vi "Four_terminal_IV_3VoltageAmp_3.1.vi"(0 "Comments":string="SA02610M.20130311\n\nall side gates=0mV\nVbg=-1V\n", 1 "Single IV curve?":bool, 2 "Experiment folder name":string="IV_test", 3 "OSC Configuration":T5(array[cluster])=[{"Signal Type"=enum."Triangle Wave", "DC"=0.00037, "Amplitude"=0.001, "frequency"=0.25, "Phase"=0.0}, {"Signal Type"=enum."Sine Wave", "DC"=0.0, "Amplitude"=0.0, "frequency"=1.0, "Phase"=0.0}, {"Signal Type"=enum."Sine Wave", "DC"=0.0, "Amplitude"=0.0, "frequency"=1.0, "Phase"=0.0}, {"Signal Type"=enum."Sine Wave", "DC"=0.0, "Amplitude"=0.0, "frequency"=1.0, "Phase"=0.0}] {"frequency" format="%0.2p"; "Amplitude" format="%0.2p"; "DC" format="%.2p"}) -> (4 "Two terminal IV":cluster{dbl[], dbl[]}(graph), 5 "I vs V":cluster{dbl[], dbl[]}[](graph), 6 "Temperature (K)":dbl=0.050002, 7 "Field (Oe)":dbl=-0.089, 8 "Connected":string="I-:4\nVbg:3\nV3+:27\nVbg:2\nV1+:28\nI+:1\nV-:5\n")   [LabVIEW 2016]
uses:
  <vilib>/DAQmx/read.llb/DAQmx Read (Analog 2D DBL NChan NSamp).vi
  <vilib>/DAQmx/write.llb/DAQmx Write (Analog 1D Wfm NChan NSamp).vi
  <userlib>/LevyLab/DAQ-Lockin-SubVI/Lockin-4461_MultiChannel - IV 3.0 globals.vi
  SubVI/ITX_Global.vi
  SubVI/PPMS Dashboard.glb.vi
  <resource>/objmgr/daqmx.rc
  <vilib>/DAQmx/configure/timing.llb/DAQmx Timing (Sample Clock).vi
  <vilib>/DAQmx/create/channels.llb/DAQmx Create Channel (AI-Voltage-Basic).vi
  <vilib>/DAQmx/configure/trigger.llb/DAQmx Start Trigger (Digital Edge).vi
  <vilib>/DAQmx/create/channels.llb/DAQmx Create Channel (AO-Voltage-Basic).vi
  <vilib>/measure/NI_MABase.lvlib
panel:
  out "phase log 2":dbl[](array[numeric])
  in  "Tab Control":T1(tab)
  out "Last Scan Image":T2(plugin-control)
  in  "File Path":path=path "C:/Experiments/2011-summer Superconductivity-Spin Hall/Device images/SA02657K_20130302.png"
  in  "PPMS      DR":bool=TRUE
  out "AI Rate":dbl=125000.0 format="%.2p"
  in  "AI Buffer Size (s)":i32=20
  in  "AI Block Size":i32=500000 format="%.0p"
  in  "AI Configuration":T3(array[cluster])=[{"AI.Coupling"=10050, "AI.Max"=10.0, "AI.Min"=-10.0, "Input physical channels"="PXI1Slot2/ai0:1"}, {"AI.Coupling"=10050, "AI.Max"=10.0, "AI.Min"=-10.0, "Input physical channels"="PXI1Slot3/ai0:1"}] {"AI.Coupling" items=["AC"=10045, "DC"=10050, "GND"=10066]}
  in  "AO Configuration":T4(array[cluster])=[{"Output physical channels"="PXI1Slot2/ao0:1", "AO. Max"=1.0, "AO.Min"=-1.0}, {"Output physical channels"="PXI1Slot3/ao0:1", "AO. Max"=10.0, "AO.Min"=-10.0}]
  in  "TIA Gain":dbl=1000000.0
  in  "Voltage Gain":dbl=100.0
  in  "decimating factor":i32=200
  in  "low cutoff freq: fl":dbl=0.1 format="%0.4f"
  in  "Daq settings":u16[](array[ring])=[0, 2, 3, 1] items=["Board 0, AI 0", "Board 0, AI 1", "Board 1, AI 0", "Board 1, AI 1"]
  out "phase log":dbl[](array[numeric])
  out "SamplesAvailable":u32[](array[numeric])=[14, 13]
  out "Sampling information":cluster{"Fs":dbl, "#s":dbl}[](array[cluster])=[{"Fs"=125000.0, "#s"=500000.0}, {"Fs"=125000.0, "#s"=500000.0}]
  out "AO Task":refnum<k21>[](array[refnum])
  out "AI task":refnum<k21>[](array[refnum])
  # "Configurations"
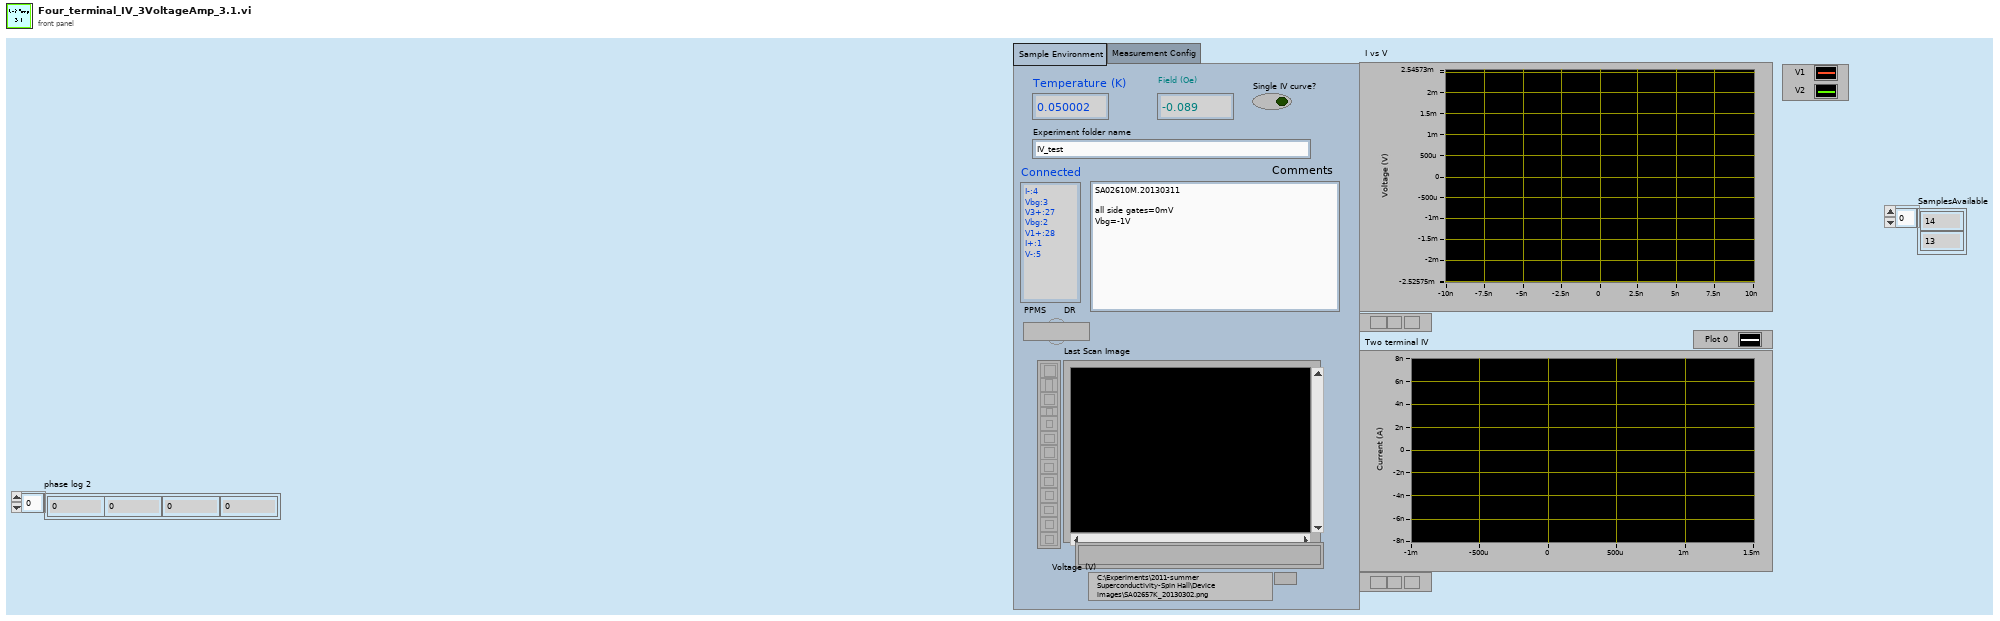
[diagram p1: front panel]
types:
  T1 = enum32{"Sample Environment", "Measurement Config"}
  T2 = typedef "IMAQ Image.ctl" = refnum<image>
  T3 = cluster{"AI.Coupling":i32, "AI.Max":dbl, "AI.Min":dbl, "Input physical channels":tag}[]
  T4 = cluster{"Output physical channels":tag, "AO. Max":dbl, "AO.Min":dbl}[]
  T5 = cluster{"Signal Type":enum16{"Sine Wave", "Triangle Wave", "Square Wave", "Sawtooth Wave"}, "DC":dbl, "Amplitude":dbl, "frequency":dbl, "Phase":dbl}[]
  T6 = cluster{"AI.Coupling":i32, "AI.Max":dbl, "AI.Min":dbl, "Input physical channels":tag}
  T7 = cluster{"Output physical channels":tag, "AO. Max":dbl, "AO.Min":dbl}
  T8 = cluster{"Signal Type":enum16{"Sine Wave", "Triangle Wave", "Square Wave", "Sawtooth Wave"}, "DC":dbl, "Amplitude":dbl, "frequency":dbl, "Phase":dbl}
  T9 = enum16{"Sine Wave", "Triangle Wave", "Square Wave", "Sawtooth Wave"}
  T10 = cluster{"Signal Type":string, "DC":string, "Amplitude":string, "frequency":string, "Phase":string}
  T11 = cluster{"Decimated Array":dbl[], "Decimated Array":dbl[]}[]
  T12 = cluster{"Decimated Array":dbl[], "Decimated Array":dbl[]}
  T13 = enum16{"Sine Wave", "Triangle Wave", "Square Wave", "Sawtooth Wave"}[]
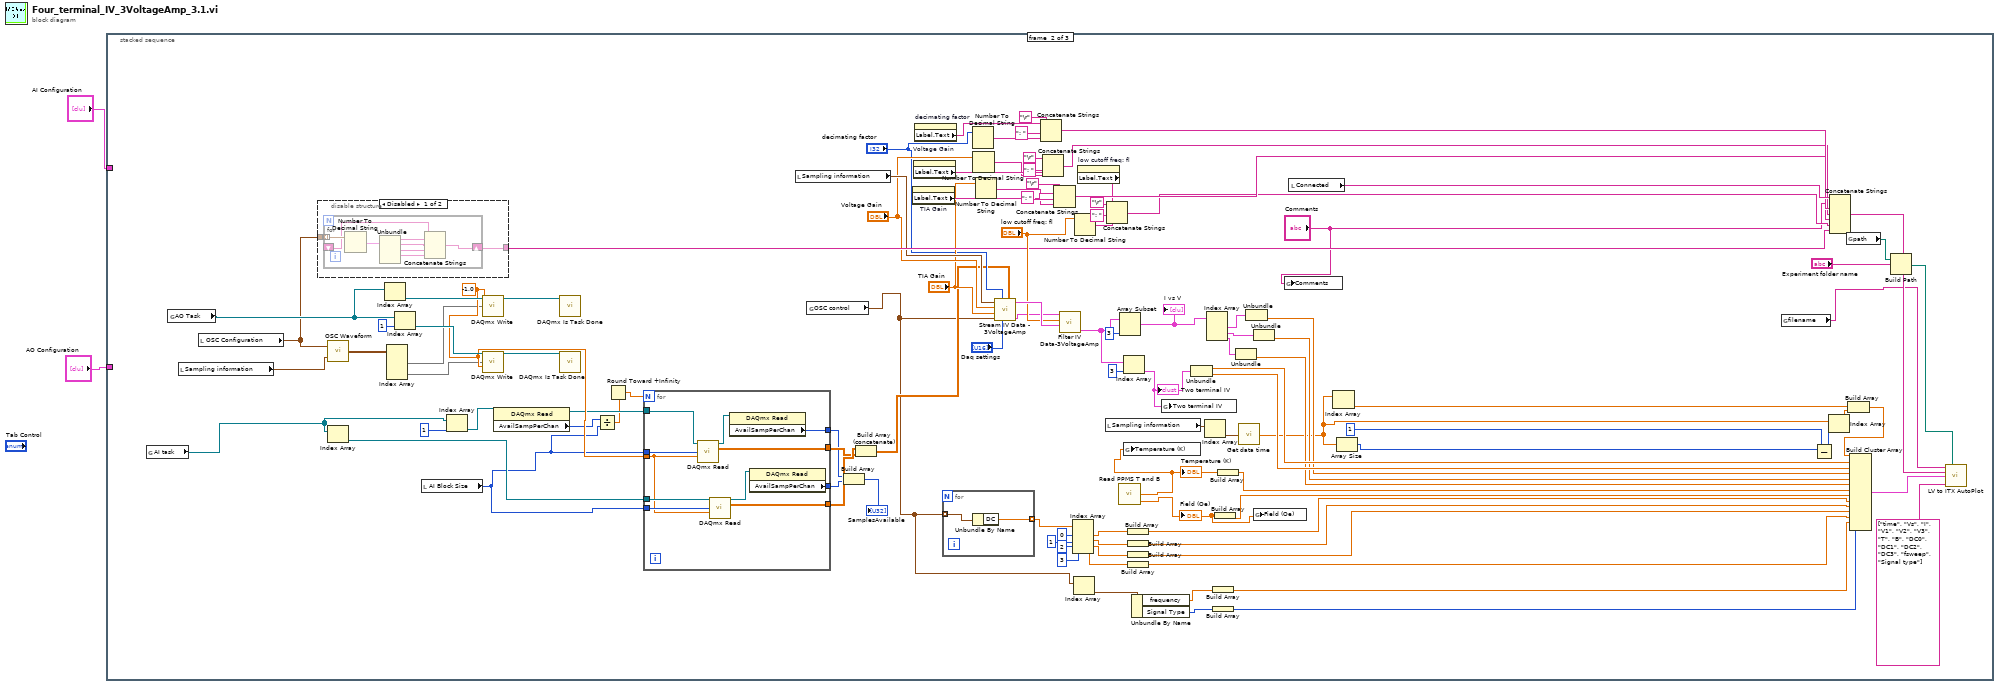
[diagram p0: block diagram]
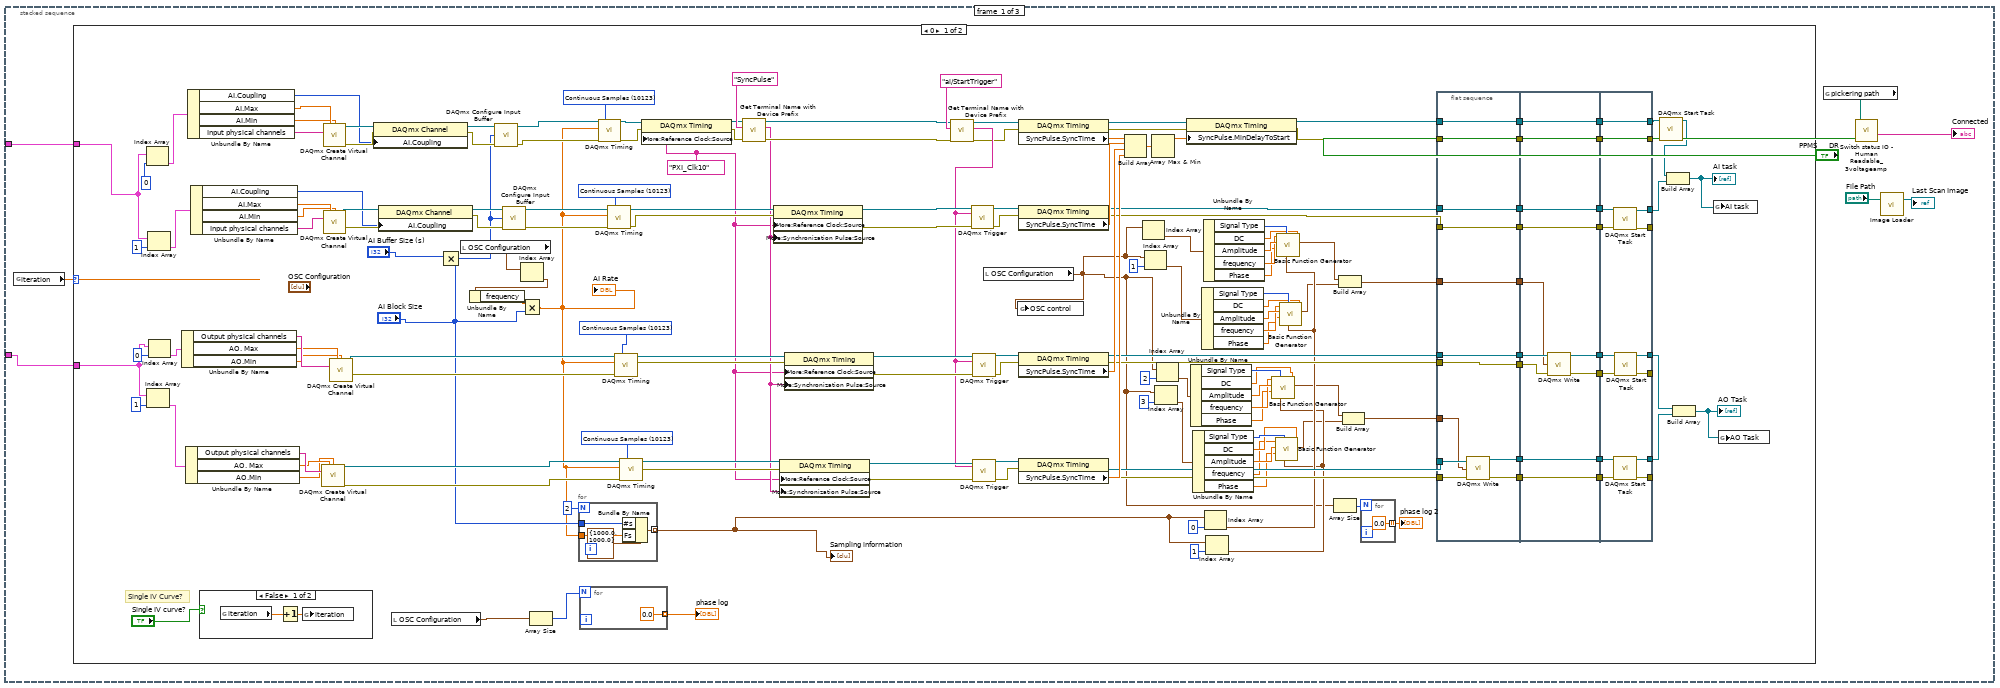
[diagram p2: hidden frame]
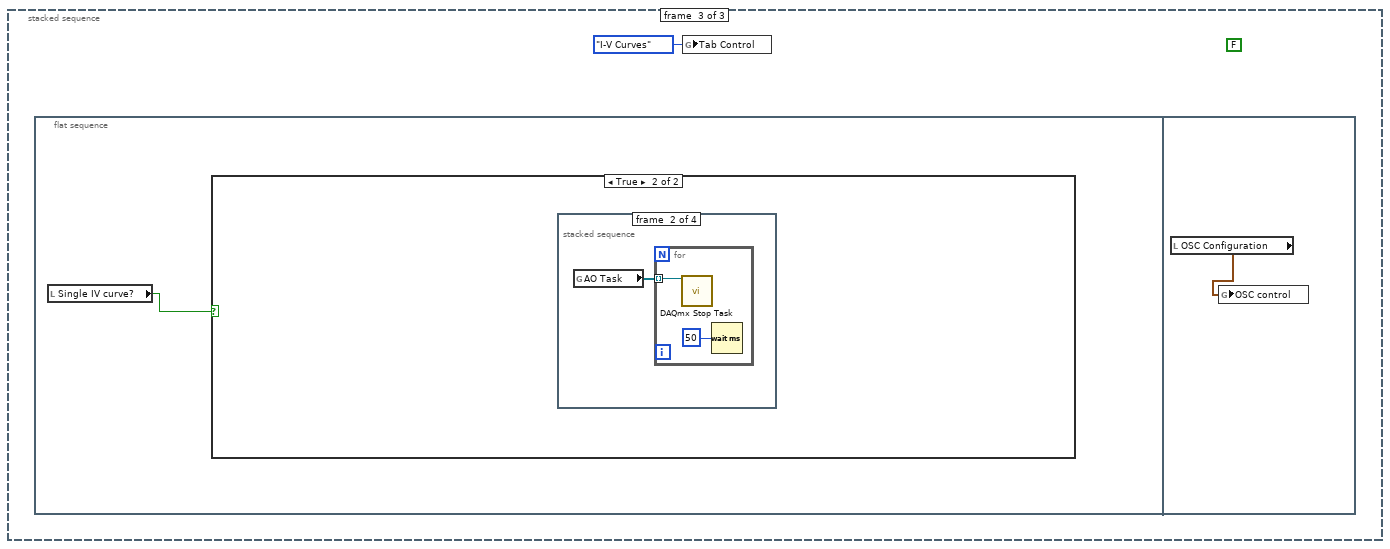
[diagram p6: hidden frame]
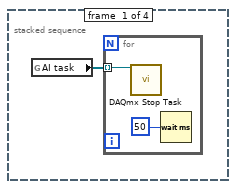
[diagram p8: hidden frame]
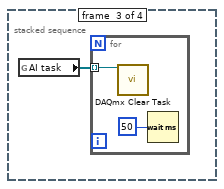
[diagram p9: hidden frame]
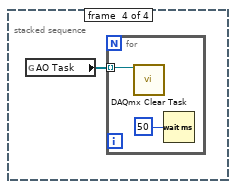
[diagram p10: hidden frame]
diagram:
  n1 = stacked-sequence {
    tunnel: "AI Configuration" -> [w4 _ _]
    tunnel: "AO Configuration" -> [w3 _ _]
    frame #0 {
      n2 = global read "Lockin-4461_MultiChannel - IV 3.0 globals.vi" "iteration"() -> (w10:dbl)
      n3 = case shown="0" w10 {
        tunnel: w4 -> [w20 _]
        tunnel: w3 -> [w19 _]
        frame 0 {
          w81 = tag "PXI_Clk10" ("RefClk.Src")
          w139 = 10123 items=["Finite Samples"=10178, "Continuous Samples"=10123] ("sample mode")
          w140 = 10123 items=["Finite Samples"=10178, "Continuous Samples"=10123] ("sample mode")
          w147 = 10123 items=["Finite Samples"=10178, "Continuous Samples"=10123] ("sample mode")
          w148 = 10123 items=["Finite Samples"=10178, "Continuous Samples"=10123] ("sample mode")
          # "Single IV Curve?"
          n4 = Index Array(array=w20, index=0) -> (element=w152:T6)
          n5 = Index Array(array=w19, index=1) -> (element=w150:T7)
          n6 = Index Array(array=w20, index=1) -> (element=w151:T6)
          n7 = Index Array(array=w19, index=0) -> (element=w149:T7)
          n8 = Unbundle By Name(w149) -> ("Output physical channels"=w90:tag, "AO. Max"=w89:dbl, "AO.Min"=w88:dbl)
          n9 = Unbundle By Name(w150) -> ("Output physical channels"=w87:tag, "AO. Max"=w86:dbl, "AO.Min"=w85:dbl)
          n10 = Unbundle By Name(w152) -> ("AI.Coupling"=w75:i32, "AI.Max"=w95:dbl, "AI.Min"=w94:dbl, "Input physical channels"=w96:tag)
          n11 = Unbundle By Name(w151) -> ("AI.Coupling"=w74:i32, "AI.Max"=w92:dbl, "AI.Min"=w91:dbl, "Input physical channels"=w93:tag)
          n12 = case shown="False" "Single IV curve?" {
            frame False {
              n13 = global read "Lockin-4461_MultiChannel - IV 3.0 globals.vi" "iteration"() -> (w223:dbl)
              n14 = Increment(x=w223) -> (x+1=w222:dbl)
              n15 = global write "Lockin-4461_MultiChannel - IV 3.0 globals.vi" "iteration"(w222) -> ()
            }
            frame True {
            }
          }
          n16 = call-poly <vilib>:"DAQmx Create Virtual Channel.vi"("maximum value"=w86, "minimum value"=w85, "physical channels"=w87) -> ("task out"=w138:refnum<k21>, "error out"=w137:errorcluster)  [unwired: 11 in]
          n17 = call-poly <vilib>:"DAQmx Create Virtual Channel.vi"("maximum value"=w95, "minimum value"=w94, "physical channels"=w96) -> ("task out"=w79:refnum<k21>, "error out"=w78:errorcluster)  [unwired: 11 in]
          n18 = call-poly <vilib>:"DAQmx Create Virtual Channel.vi"("maximum value"=w92, "minimum value"=w91, "physical channels"=w93) -> ("task out"=w77:refnum<k21>, "error out"=w76:errorcluster)  [unwired: 11 in]
          n19 = call-poly <vilib>:"DAQmx Create Virtual Channel.vi"("maximum value"=w89, "minimum value"=w88, "physical channels"=w90) -> ("task out"=w98:refnum<k21>, "error out"=w97:errorcluster)  [unwired: 11 in]
          n20 = property class="DAQmx Channel"(reference=w79, error in=w78, "AI.Coupling"=w75) -> (reference out=w73:refnum<k21>, error out=w72:errorcluster)
          n21 = property class="DAQmx Channel"(reference=w77, error in=w76, "AI.Coupling"=w74) -> (reference out=w71:refnum<k21>, error out=w70:errorcluster)
          n22 = local read "OSC Configuration"() -> (w176:T5)
          n23 = Multiply(x="AI Buffer Size (s)", y="AI Block Size") -> (x*y=w65:i32)
          n24 = local read "OSC Configuration"() -> (w16:T5)
          n25 = call <vilib>:"DAQmx Configure Input Buffer.vi"("task/channels in"=w73, "buffer size (in samples per channel)"=w65, "error in"=w72) -> ("task out"=w69:refnum<k21>, "error out"=w68:errorcluster)  [unwired: 11 in]
          n26 = call <vilib>:"DAQmx Configure Input Buffer.vi"("task/channels in"=w71, "buffer size (in samples per channel)"=w65, "error in"=w70) -> ("task out"=w67:refnum<k21>, "error out"=w66:errorcluster)  [unwired: 11 in]
          n27 = Index Array(array=w16) -> (element=w25:T8)  [unwired: 1 in]
          n28 = Unbundle By Name(w25) -> ("frequency"=w24:dbl)
          n29 = Multiply(x=w24, y="AI Block Size") -> (x*y=w15:dbl)
          "AI Rate" <- w15
          n30 = Array Size(array=w176) -> (size(s)=w178:i32)
          n31 = for {
            N: 2 -> [_]
            tunnel: w15 -> [w183]
            tunnel: "AI Block Size" -> [w182]
            tunnel: [w180] -> w12 mode=indexing
            n32 = Bundle By Name(cluster=cluster{"Fs":dbl, "#s":dbl} {"Fs"=1000.0, "#s"=1000.0} ("sampling info"), "#s"=w182, "Fs"=w183) -> (w180:cluster{"Fs":dbl, "#s":dbl})
          }
          "Sampling information" <- w12
          n33 = for {
            N: w178 -> [_]
            tunnel: [0.0] -> w179 mode=indexing
          }
          "phase log" <- w179
          n34 = call-poly <vilib>:"DAQmx Timing.vi"("task/channels in"=w69, "sample mode"=w148, "rate"=w15, "error in"=w68) -> ("task out"=w142:refnum<k21>, "error out"=w141:errorcluster)  [unwired: 10 in]
          n35 = call-poly <vilib>:"DAQmx Timing.vi"("task/channels in"=w67, "sample mode"=w147, "rate"=w15, "error in"=w66) -> ("task out"=w144:refnum<k21>, "error out"=w143:errorcluster)  [unwired: 10 in]
          n36 = call-poly <vilib>:"DAQmx Timing.vi"("task/channels in"=w98, "sample mode"=w140, "rate"=w15, "error in"=w97) -> ("task out"=w135:refnum<k21>, "error out"=w134:errorcluster)  [unwired: 10 in]
          n37 = call-poly <vilib>:"DAQmx Timing.vi"("task/channels in"=w138, "sample mode"=w139, "rate"=w15, "error in"=w137) -> ("task out"=w136:refnum<k21>, "error out"=w131:errorcluster)  [unwired: 10 in]
          n38 = property class="DAQmx Timing"(reference=w142, error in=w141, "More:Reference Clock:Source"=w81) -> (reference out=w82:refnum<k21>, error out=w80:errorcluster)
          n39 = call "Get Terminal Name with Device Prefix.vi"("error in (no error)"=w80, "Local Terminal Name"="SyncPulse", "task/channels in"=w82) -> ("error out"=w124:errorcluster, "Terminal Name with Device Prefix"=w83:tag, "task out"=w125:refnum<k21>)  [unwired: 6 in]
          n40 = property class="DAQmx Timing"(reference=w144, error in=w143, "More:Reference Clock:Source"=w81, "More:Synchronization Pulse:Source"=w83) -> (reference out=w146:refnum<k21>, error out=w145:errorcluster)
          n41 = property class="DAQmx Timing"(reference=w136, error in=w131, "More:Reference Clock:Source"=w81, "More:Synchronization Pulse:Source"=w83) -> (reference out=w128:refnum<k21>, error out=w127:errorcluster)
          n42 = property class="DAQmx Timing"(reference=w135, error in=w134, "More:Reference Clock:Source"=w81, "More:Synchronization Pulse:Source"=w83) -> (reference out=w130:refnum<k21>, error out=w129:errorcluster)
          n43 = call "Get Terminal Name with Device Prefix.vi"("error in (no error)"=w124, "Local Terminal Name"="ai/StartTrigger", "task/channels in"=w125) -> ("error out"=w121:errorcluster, "Terminal Name with Device Prefix"=w123:tag, "task out"=w122:refnum<k21>)  [unwired: 6 in]
          n44 = call-poly <vilib>:"DAQmx Trigger.vi"("task/channels in"=w146, "source"=w123, "error in"=w145) -> ("task out"=w117:refnum<k21>, "error out"=w118:errorcluster)  [unwired: 11 in]
          n45 = call-poly <vilib>:"DAQmx Trigger.vi"("task/channels in"=w130, "source"=w123, "error in"=w129) -> ("task out"=w115:refnum<k21>, "error out"=w116:errorcluster)  [unwired: 11 in]
          n46 = call-poly <vilib>:"DAQmx Trigger.vi"("task/channels in"=w128, "source"=w123, "error in"=w127) -> ("task out"=w120:refnum<k21>, "error out"=w119:errorcluster)  [unwired: 11 in]
          n47 = local read "OSC Configuration"() -> (w11:T5)
          n48 = global write "Lockin-4461_MultiChannel - IV 3.0 globals.vi" "OSC control"(w11) -> ()
          n49 = property class="DAQmx Timing"(reference=w122, error in=w121) -> (reference out=w112:refnum<k21>, error out=w113:errorcluster, "SyncPulse.SyncTime"=w114:dbl)
          n50 = property class="DAQmx Timing"(reference=w117, error in=w118) -> (reference out=w103:refnum<k21>, error out=w104:errorcluster, "SyncPulse.SyncTime"=w109:dbl)
          n51 = property class="DAQmx Timing"(reference=w115, error in=w116) -> (reference out=w101:refnum<k21>, error out=w102:errorcluster, "SyncPulse.SyncTime"=w108:dbl)
          n52 = property class="DAQmx Timing"(reference=w120, error in=w119) -> (reference out=w99:refnum<k21>, error out=w100:errorcluster, "SyncPulse.SyncTime"=w107:dbl)
          n53 = Build Array(w114, w109, w108, w107) -> (w111:dbl[])
          n54 = Index Array(array=w11) -> (element=w62:T8)  [unwired: 1 in]
          n55 = Index Array(array=w11, index=1) -> (element=w61:T8)
          n56 = Array Max & Min(array=w111) -> (max value=w110:dbl)  [unwired: 3 out]
          n57 = Index Array(array=w11, index=3) -> (element=w60:T8)
          n58 = Index Array(array=w11, index=2) -> (element=w63:T8)
          n59 = property class="DAQmx Timing"(reference=w112, error in=w113, "SyncPulse.MinDelayToStart"=w110) -> (reference out=w105:refnum<k21>, error out=w106:errorcluster)
          n60 = Unbundle By Name(w63) -> ("Signal Type"=w49:T9, "DC"=w48:dbl, "Amplitude"=w47:dbl, "frequency"=w46:dbl, "Phase"=w45:dbl)
          n61 = Unbundle By Name(w60) -> ("Signal Type"=w44:T9, "DC"=w43:dbl, "Amplitude"=w42:dbl, "frequency"=w41:dbl, "Phase"=w40:dbl)
          n62 = Unbundle By Name(w61) -> ("Signal Type"=w54:T9, "DC"=w53:dbl, "Amplitude"=w52:dbl, "frequency"=w51:dbl, "Phase"=w50:dbl)
          n63 = Unbundle By Name(w62) -> ("Signal Type"=w59:T9, "DC"=w58:dbl, "Amplitude"=w57:dbl, "frequency"=w56:dbl, "Phase"=w55:dbl)
          n64 = Index Array(array=w12, index=0) -> (element=w37:cluster{"Fs":dbl, "#s":dbl})
          n65 = Index Array(array=w12, index=1) -> (element=w36:cluster{"Fs":dbl, "#s":dbl})
          n66 = call <vilib>:"Basic Function Generator.vi"("offset"=w48, "sampling info"=w36, "signal type"=w49, "phase"=w45, "amplitude"=w47, "frequency"=w46) -> ("signal out"=w32:waveform(dbl))  [unwired: 3 in, 2 out]
          n67 = call <vilib>:"Basic Function Generator.vi"("offset"=w43, "sampling info"=w36, "signal type"=w44, "phase"=w40, "amplitude"=w42, "frequency"=w41) -> ("signal out"=w31:waveform(dbl))  [unwired: 3 in, 2 out]
          n68 = call <vilib>:"Basic Function Generator.vi"("offset"=w58, "sampling info"=w37, "signal type"=w59, "phase"=w55, "amplitude"=w57, "frequency"=w56) -> ("signal out"=w35:waveform(dbl))  [unwired: 3 in, 2 out]
          n69 = call <vilib>:"Basic Function Generator.vi"("offset"=w53, "sampling info"=w37, "signal type"=w54, "phase"=w50, "amplitude"=w52, "frequency"=w51) -> ("signal out"=w34:waveform(dbl))  [unwired: 3 in, 2 out]
          n70 = Array Size(array=w11) -> (size(s)=w157:i32)
          n71 = Build Array(w35, w34) -> (w33:waveform(dbl)[])
          n72 = Build Array(w32, w31) -> (w30:waveform(dbl)[])
          n73 = for {
            N: w157 -> [_]
            tunnel: [0.0] -> w158 mode=indexing
          }
          "phase log 2" <- w158
          n74 = flat-sequence {
            tunnel: w106 -> [w192]
            tunnel: w105 -> [w193]
            tunnel: w104 -> [w194]
            tunnel: w103 -> [w195]
            tunnel: [w195] -> w175
            tunnel: [w194] -> w174
            tunnel: [w193] -> w173
            tunnel: [w192] -> w172
            tunnel: [w191] -> w171
            tunnel: w102 -> [w191]
            tunnel: [w190] -> w170
            tunnel: w101 -> [w190]
            tunnel: w100 -> [w189]
            tunnel: w99 -> [w188]
            tunnel: [w187] -> w169
            tunnel: [w186] -> w168
            tunnel: w33 -> [w185]
            tunnel: [w185] -> w167
            tunnel: w30 -> [w184]
            tunnel: [w206] -> w166
            tunnel: [w205] -> w165
            tunnel: [w204] -> w164
            tunnel: [w203] -> w163
            tunnel: w175 -> [w206]
            tunnel: w174 -> [w205]
            tunnel: w173 -> [w204]
            tunnel: w172 -> [w203]
            tunnel: w171 -> [w202]
            tunnel: w170 -> [w201]
            tunnel: [w200] -> w162
            tunnel: w169 -> [w200]
            tunnel: [w199] -> w161
            tunnel: w168 -> [w199]
            tunnel: [w198] -> w160
            tunnel: [w197] -> w159
            tunnel: w167 -> [w196]
            tunnel: [w213] -> _
            tunnel: [w214] -> w27
            tunnel: [w215] -> _
            tunnel: [w216] -> w26
            tunnel: [w217] -> _
            tunnel: [w219] -> w28
            tunnel: [w212] -> w133
            tunnel: [w211] -> w132
            tunnel: w166 -> [w220]
            tunnel: w165 -> [w218]
            tunnel: w164 -> [w212]
            tunnel: w163 -> [w211]
            tunnel: w162 -> [w210]
            tunnel: w161 -> [w209]
            tunnel: w160 -> [w208]
            tunnel: w159 -> [w207]
            frame #0 {
              n75 = call-poly <vilib>:"DAQmx Write.vi"("task/channels in"=w188, "data"=w184, "error in"=w189) -> ("task out"=w186:refnum<k21>, "error out"=w187:errorcluster)  [unwired: 10 in, 1 out]
            }
            frame #1 {
              n76 = call-poly <vilib>:"DAQmx Write.vi"("task/channels in"=w201, "data"=w196, "error in"=w202) -> ("task out"=w197:refnum<k21>, "error out"=w198:errorcluster)  [unwired: 10 in, 1 out]
            }
            frame #2 {
              n77 = call <vilib>:"DAQmx Start Task.vi"("task/channels in"=w220, "error in"=w218) -> ("task out"=w219:refnum<k21>, "error out"=w217:errorcluster)  [unwired: 12 in]
              n78 = call <vilib>:"DAQmx Start Task.vi"("task/channels in"=w209, "error in"=w210) -> ("task out"=w216:refnum<k21>, "error out"=w215:errorcluster)  [unwired: 12 in]
              n79 = call <vilib>:"DAQmx Start Task.vi"("task/channels in"=w207, "error in"=w208) -> ("task out"=w214:refnum<k21>, "error out"=w213:errorcluster)  [unwired: 12 in]
            }
          }
          n80 = call <vilib>:"DAQmx Start Task.vi"("task/channels in"=w133, "error in"=w132) -> ("task out"=w29:refnum<k21>)  [unwired: 12 in, 1 out]
          n81 = Build Array(w29, w28) -> (w14:refnum<k21>[])
          "AI task" <- w14
          n82 = Build Array(w27, w26) -> (w13:refnum<k21>[])
          "AO Task" <- w13
          n83 = global write "Lockin-4461_MultiChannel - IV 3.0 globals.vi" "AI task"(w14) -> ()
          n84 = global write "Lockin-4461_MultiChannel - IV 3.0 globals.vi" "AO Task"(w13) -> ()
        }
        frame 1, Default {
        }
      }
      n85 = global read "ITX_Global.vi" "pickering path"() -> (w7:path)
      n86 = call <userlib>:"Switch status IO - Human Readable_3voltageamp.vi"("PPMS      DR"="PPMS      DR", "Switch status"=w7) -> ("String"=→"Connected":string)  [unwired: 2 in]
      n87 = call "Image Loader.vi"("File Path"="File Path") -> ("Last Scan Image"=→"Last Scan Image":T2)  [unwired: 2 in]
    }
    frame #1 {
      w321 = -1.0 ("timeout")
      n88 = global read "Lockin-4461_MultiChannel - IV 3.0 globals.vi" "AI task"() -> (w332:refnum<k21>[])
      n89 = global read "Lockin-4461_MultiChannel - IV 3.0 globals.vi" "AO Task"() -> (w292:refnum<k21>[])
      n90 = local read "Sampling information"() -> (w334:cluster{"Fs":dbl, "#s":dbl}[])
      n91 = local read "OSC Configuration"() -> (w227:T5)
      n92 = disable-structure shown="Disabled" {
        disable-tunnel: w227 -> [w349 _]
        disable-tunnel: [w348 _] -> w318
        frame Disabled {
          n93 = for {
            tunnel: w349 -> [w357] mode=indexing
            shift-right: [w351] -> w348
            shift-left: _ -> [w350]
            n94 = Number To Decimal String(number=w357) -> (decimal integer string=w356:T10)  [unwired: 1 in]
            n95 = Unbundle(w356) -> ("Signal Type"=w355:string, "DC"=w354:string, "Amplitude"=w353:string, "frequency"=w352:string)  [unwired: 1 out]
            n96 = Concatenate Strings(w350, w355, w354, w353, w352) -> (w351:string)
          }
        }
        frame Enabled {
        }
      }
      n97 = call "OSC Waveform.vi"("Sampling information"=w334, "OSC Configuration"=w227) -> ("OSC Waveforms"=w327:waveform(dbl)[][])
      n98 = Index Array(array=w332) -> (element=w331:refnum<k21>)  [unwired: 1 in]
      n99 = Index Array(array=w292) -> (element=w326:refnum<k21>)  [unwired: 1 in]
      n100 = Index Array(array=w327) -> (element #1=w290:waveform(dbl)[], element #2=w291:waveform(dbl)[])  [unwired: 4 in]
      n101 = Index Array(array=w292, index=1) -> (element=w324:refnum<k21>)
      n102 = local read "AI Block Size"() -> (w229:i32)
      n103 = Index Array(array=w332, index=1) -> (element=w238:refnum<k21>)
      n104 = call-poly <vilib>:"DAQmx Write.vi"("task/channels in"=w326, "data"=w290, "timeout"=w321) -> ("task out"=w329:refnum<k21>)  [unwired: 10 in, 2 out]
      n105 = call-poly <vilib>:"DAQmx Write.vi"("task/channels in"=w324, "data"=w291, "timeout"=w321) -> ("task out"=w328:refnum<k21>)  [unwired: 10 in, 2 out]
      n106 = property class="DAQmx Read"(reference=w238) -> (reference out=w237:refnum<k21>, "AvailSampPerChan"=w236:u32)  [unwired: 1 in, 1 out]
      n107 = call <vilib>:"DAQmx Is Task Done.vi"("task/channels in"=w329) -> ()  [unwired: 12 in, 3 out]
      n108 = call <vilib>:"DAQmx Is Task Done.vi"("task/channels in"=w328) -> ()  [unwired: 12 in, 3 out]
      n109 = Divide(x=w236, y=w229) -> (x/y=w235:dbl)
      n110 = Round Toward +Infinity(x=w235) -> (ceil(x): smallest int >= x=w228:dbl)
      n111 = for {
        N: w228 -> [_]
        tunnel: w331 -> [w345]
        tunnel: [w344] -> w323
        tunnel: w229 -> [w343]
        tunnel: [w342] -> w322
        tunnel: w321 -> [w341]
        tunnel: w237 -> [w340]
        tunnel: w229 -> [w339]
        tunnel: [w336] -> w234
        tunnel: [w335] -> w233
        n112 = call-poly <vilib>:"DAQmx Read.vi"("task/channels in"=w340, "number of samples per channel"=w339, "timeout"=w341) -> ("task out"=w338:refnum<k21>, "data"=w342:dbl[][])  [unwired: 10 in, 1 out]
        n113 = call-poly <vilib>:"DAQmx Read.vi"("task/channels in"=w345, "number of samples per channel"=w343, "timeout"=w341) -> ("task out"=w337:refnum<k21>, "data"=w344:dbl[][])  [unwired: 10 in, 1 out]
        n114 = property class="DAQmx Read"(reference=w338) -> ("AvailSampPerChan"=w336:u32)  [unwired: 1 in, 2 out]
        n115 = property class="DAQmx Read"(reference=w337) -> ("AvailSampPerChan"=w335:u32)  [unwired: 1 in, 2 out]
      }
      n116 = local read "Sampling information"() -> (w297:cluster{"Fs":dbl, "#s":dbl}[])
      n117 = global read "Lockin-4461_MultiChannel - IV 3.0 globals.vi" "OSC control"() -> (w226:T5)
      n118 = Build Array(w234, w233) -> (→"SamplesAvailable":u32[])
      n119 = Build Array (concatenate)(w323, w322) -> (w293:dbl[][])
      n120 = property on="TIA Gain" class="DigNum (strict)"() -> ("Label.Text"=w304:string)  [unwired: 2 in, 2 out]
      n121 = property on="Voltage Gain" class="DigNum (strict)"() -> ("Label.Text"=w311:string)  [unwired: 2 in, 2 out]
      n122 = property on="decimating factor" class="DigNum (strict)"() -> ("Label.Text"=w307:string)  [unwired: 2 in, 2 out]
      n123 = for {
        tunnel: w226 -> [w347] mode=indexing
        tunnel: [w346] -> w262 mode=indexing
        n124 = Unbundle By Name(w347) -> ("DC"=w346:dbl)
      }
      n125 = Number To Decimal String(number="decimating factor") -> (decimal integer string=w306:string)  [unwired: 1 in]
      n126 = Number To Decimal String(number="Voltage Gain") -> (decimal integer string=w310:string)  [unwired: 1 in]
      n127 = Number To Decimal String(number="TIA Gain") -> (decimal integer string=w303:string)  [unwired: 1 in]
      n128 = call "Stream IV Data - 3VoltageAmp.vi"("Input signal"=w293, "Daq settings"="Daq settings", "decimating factor"="decimating factor", "OSC Configuration"=w226, "TIA Gain"="TIA Gain", "Voltage Gain"="Voltage Gain", "Sampling information"=w297) -> ("Four terminal IVs"=w286:T11, "Two terminal IV"=w333:T12)  [unwired: 3 in]
      n129 = Concatenate Strings("\r" ("string"), w307, ": " ("string"), w306) -> (w317:string)
      n130 = Concatenate Strings("\r" ("string"), w311, ": " ("string"), w310) -> (w316:string)
      n131 = Concatenate Strings("\r" ("string"), w304, ": " ("string"), w303) -> (w315:string)
      n132 = call "Filter IV Data-3VoltageAmp.vi"("Two terminal IV"=w333, "low cutoff freq: fl"="low cutoff freq: fl", "Four terminal IVs"=w286) -> ("V vs I 2"=w285:cluster{dbl[], dbl[]}[])
      n133 = Index Array(array=w262, index #1=0 ("index"), index #2=1 ("index"), index #3=2 ("index"), index #4=3 ("index")) -> (element #1=w257:dbl, element #2=w256:dbl, element #3=w255:dbl, element #4=w254:dbl)
      n134 = Index Array(array=w226) -> (element=w249:T8)  [unwired: 1 in]
      n135 = Number To Decimal String(number="low cutoff freq: fl") -> (decimal integer string=w299:string)  [unwired: 1 in]
      n136 = property on="low cutoff freq: fl" class="DigNum (strict)"() -> ("Label.Text"=w300:string)  [unwired: 2 in, 2 out]
      n137 = local read "Sampling information"() -> (w273:cluster{"Fs":dbl, "#s":dbl}[])
      n138 = Concatenate Strings("\r" ("string"), w300, ": " ("string"), w299) -> (w314:string)
      n139 = call "Read PPMS T and B.vi"() -> ("Field"=w241:dbl, "Temperature"=w242:dbl)  [unwired: 3 in, 1 out]
      "Temperature (K)" <- w242
      "Field (Oe)" <- w241
      n140 = Array Subset(array=w285, length=3) -> (w279:cluster{dbl[], dbl[]}[])  [unwired: 1 in]
      "I vs V" <- w279
      n141 = Index Array(array=w285, index=3) -> (element=w240:cluster{dbl[], dbl[]})
      "Two terminal IV" <- w240
      n142 = global write "PPMS Dashboard.glb.vi" "Temperature (K)"(w242) -> ()
      n143 = Build Array(w257) -> (w253:dbl[])
      n144 = Build Array(w256) -> (w252:dbl[])
      n145 = Build Array(w255) -> (w251:dbl[])
      n146 = Build Array(w254) -> (w250:dbl[])
      n147 = Unbundle By Name(w249) -> ("frequency"=w248:dbl, "Signal Type"=w231:T9)
      n148 = global write "PPMS Dashboard.glb.vi" "Two terminal IV"(w240) -> ()
      n149 = Unbundle(w240) -> (w281:dbl[], w280:dbl[])
      n150 = Index Array(array=w273) -> (element=w272:cluster{"Fs":dbl, "#s":dbl})  [unwired: 1 in]
      n151 = Index Array(array=w279) -> (element #1=w270:cluster{dbl[], dbl[]}, element #2=w278:cluster{dbl[], dbl[]}, element #3=w277:cluster{dbl[], dbl[]})  [unwired: 3 in]
      n152 = Build Array(w248) -> (w247:dbl[])
      n153 = Build Array(w231) -> (w230:T13)
      n154 = Build Array(w241) -> (w283:dbl[])
      n155 = Build Array(w242) -> (w282:dbl[])
      n156 = Unbundle(w277) -> (w276:dbl[])  [unwired: 1 out]
      n157 = call "Get data time.vi"("sampling info"=w272) -> ("Array"=w269:dbl[])
      n158 = Unbundle(w270) -> (w274:dbl[])  [unwired: 1 out]
      n159 = Unbundle(w278) -> (w275:dbl[])  [unwired: 1 out]
      n160 = global write "PPMS Dashboard.glb.vi" "Field (Oe)"(w241) -> ()
      n161 = global write "PPMS Dashboard.glb.vi" "Comments"("Comments") -> ()
      n162 = local read "Connected"() -> (w320:string)
      n163 = Index Array(array=w269) -> (element=w268:dbl)  [unwired: 1 in]
      n164 = Array Size(array=w269) -> (size(s)=w265:i32)
      n165 = global read "ITX_Global.vi" "filename"() -> (w225:string)
      n166 = Subtract(x=w265, y=1) -> (x-y=w263:i32)
      n167 = Index Array(array=w269, index=w263) -> (element=w267:dbl)
      n168 = Concatenate Strings(w320, "Comments", w317, w316, w315, w314, w318) -> (w271:string)
      n169 = global read "ITX_Global.vi" "path"() -> (w245:path)
      n170 = Build Array(w268, w267) -> (w266:dbl[])
      n171 = Build Cluster Array(w266, w281, w280, w274, w275, w276, w282, w283, w253, w252, w251, w250, w247, w230) -> (w284:cluster{dbl[]}[])
      n172 = Build Path(base path=w245, name or relative path="Experiment folder name") -> (appended path=w244:path)
      n173 = call <userlib>:"LV to ITX AutoPlot.vi"("filename"=w225, "path"=w244, "Notes"=w271, "Data"=w284, "wavenames (.Vx, etc)"=string[] ["time", "Vs", "I", "V1", "V2", "V3", "T", "B", "DC0", "DC1", "DC2", "DC3", "fsweep", "Signal type"]) -> ()  [unwired: 10 in, 1 out]
    }
    frame #2 {
      (unwired) FALSE
      n174 = flat-sequence {
        frame #0 {
          n175 = local read "Single IV curve?"() -> (w359:bool)
          n176 = case shown="True" w359 {
            frame False {
            }
            frame True {
              n177 = stacked-sequence {
                frame #0 {
                  n178 = global read "Lockin-4461_MultiChannel - IV 3.0 globals.vi" "AI task"() -> (w360:refnum<k21>[])
                  n179 = for {
                    tunnel: w360 -> [w362] mode=indexing
                    n180 = call <vilib>:"DAQmx Stop Task.vi"("task/channels in"=w362) -> ()  [unwired: 13 in, 2 out]
                    n181 = Wait (ms)(milliseconds to wait=u32 50) -> ()  [unwired: 1 out]
                  }
                }
                frame #1 {
                  n182 = global read "Lockin-4461_MultiChannel - IV 3.0 globals.vi" "AO Task"() -> (w363:refnum<k21>[])
                  n183 = for {
                    tunnel: w363 -> [w365] mode=indexing
                    n184 = call <vilib>:"DAQmx Stop Task.vi"("task/channels in"=w365) -> ()  [unwired: 13 in, 2 out]
                    n185 = Wait (ms)(milliseconds to wait=u32 50) -> ()  [unwired: 1 out]
                  }
                }
                frame #2 {
                  n186 = global read "Lockin-4461_MultiChannel - IV 3.0 globals.vi" "AI task"() -> (w366:refnum<k21>[])
                  n187 = for {
                    tunnel: w366 -> [w368] mode=indexing
                    n188 = call <vilib>:"DAQmx Clear Task.vi"("task in"=w368) -> ()  [unwired: 14 in, 1 out]
                    n189 = Wait (ms)(milliseconds to wait=u32 50) -> ()  [unwired: 1 out]
                  }
                }
                frame #3 {
                  n190 = global read "Lockin-4461_MultiChannel - IV 3.0 globals.vi" "AO Task"() -> (w369:refnum<k21>[])
                  n191 = for {
                    tunnel: w369 -> [w371] mode=indexing
                    n192 = call <vilib>:"DAQmx Clear Task.vi"("task in"=w371) -> ()  [unwired: 14 in, 1 out]
                    n193 = Wait (ms)(milliseconds to wait=u32 50) -> ()  [unwired: 1 out]
                  }
                }
              }
            }
          }
        }
        frame #1 {
          n194 = local read "OSC Configuration"() -> (w372:T5)
          n195 = global write "Lockin-4461_MultiChannel - IV 3.0 globals.vi" "OSC control"(w372) -> ()
        }
      }
      n196 = global write "PPMS Dashboard.glb.vi" "Tab Control"(enum32{"I-V Curves", "Cooldown/Warmup"}."I-V Curves" ("Tab Control")) -> ()
    }
  }
